vi "Power ON-Ganging.vi"(8 "error in":errorcluster, 11 "Power ON":T1={"Master/single Resource name"="", "Slave resource name"=[], "System configuration"=enum."Parallel", "Output function"=1006, "Voltage/current level"=0.0, "Voltage/current limit"=0.0, "Sense"=1009} {"Output function" items=["DC Voltage"=1006, "DC Current"=1007, "Pulse Voltage"=1049, "Pulse Current"=1050]; "Sense" items=["Local"=1008, "Remote"=1009]}) -> (0 "error out":errorcluster, 3 "Status":string)   [LabVIEW 2021]
doc: "This VI will configure the source device to DC Current or DC Voltage mode to ower on the DUT for ganged or stacked channel configuration."
uses:
  controls/Power ON-Ganging.ctl
  <instrlib>/niDCPower/nidcpower.llb/niDCPower Source Mode.ctl
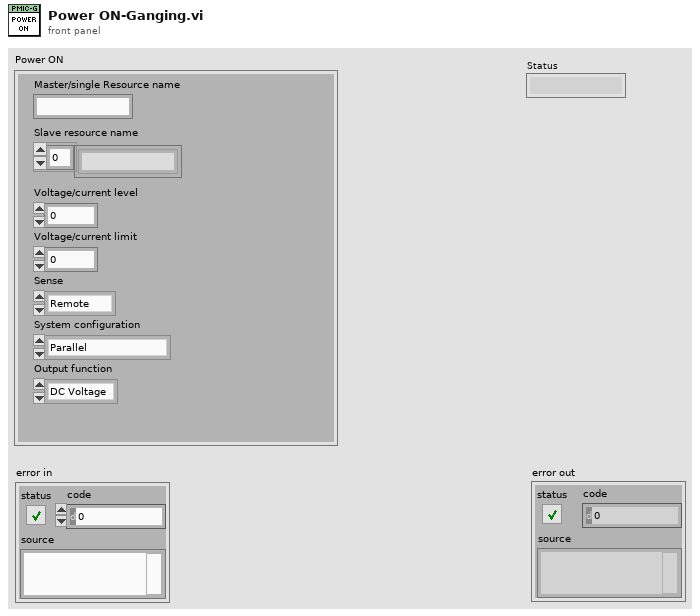
[diagram p1: front panel]
types:
  T1 = typedef "Power ON-Ganging.ctl" = cluster{"Master/single Resource name":string, "Slave resource name":string[], "System configuration":enum32{"Series", "Parallel", "Manual"}, "Output function":i32, "Voltage/current level":dbl, "Voltage/current limit":dbl, "Sense":i32}
  T2 = typedef "niDCPower Source Mode.ctl" = i32
  T3 = typedef "NIDCPower_channel_ganging - ctl - channel def.ctl" = cluster{"resource name":refnum<k15>, "channels":string, "Channel Mode":T4}
  T4 = typedef "NIDCPower_channel_ganging - ctl - channel mode.ctl" = enum32{"Master", "Slave", "Slave - Inverted"}
  T5 = typedef "NIDCPower_channel_ganging - ctl - ganged session.ctl" = cluster{"Ganged Config":T6, "Session List":refnum<k15>[], "Session Mode":T4[], "Channel":string[]}
  T6 = typedef "NIDCPower_channel_ganging - ctl - ganged config.ctl" = enum32{"Series", "Parallel", "Manual"}
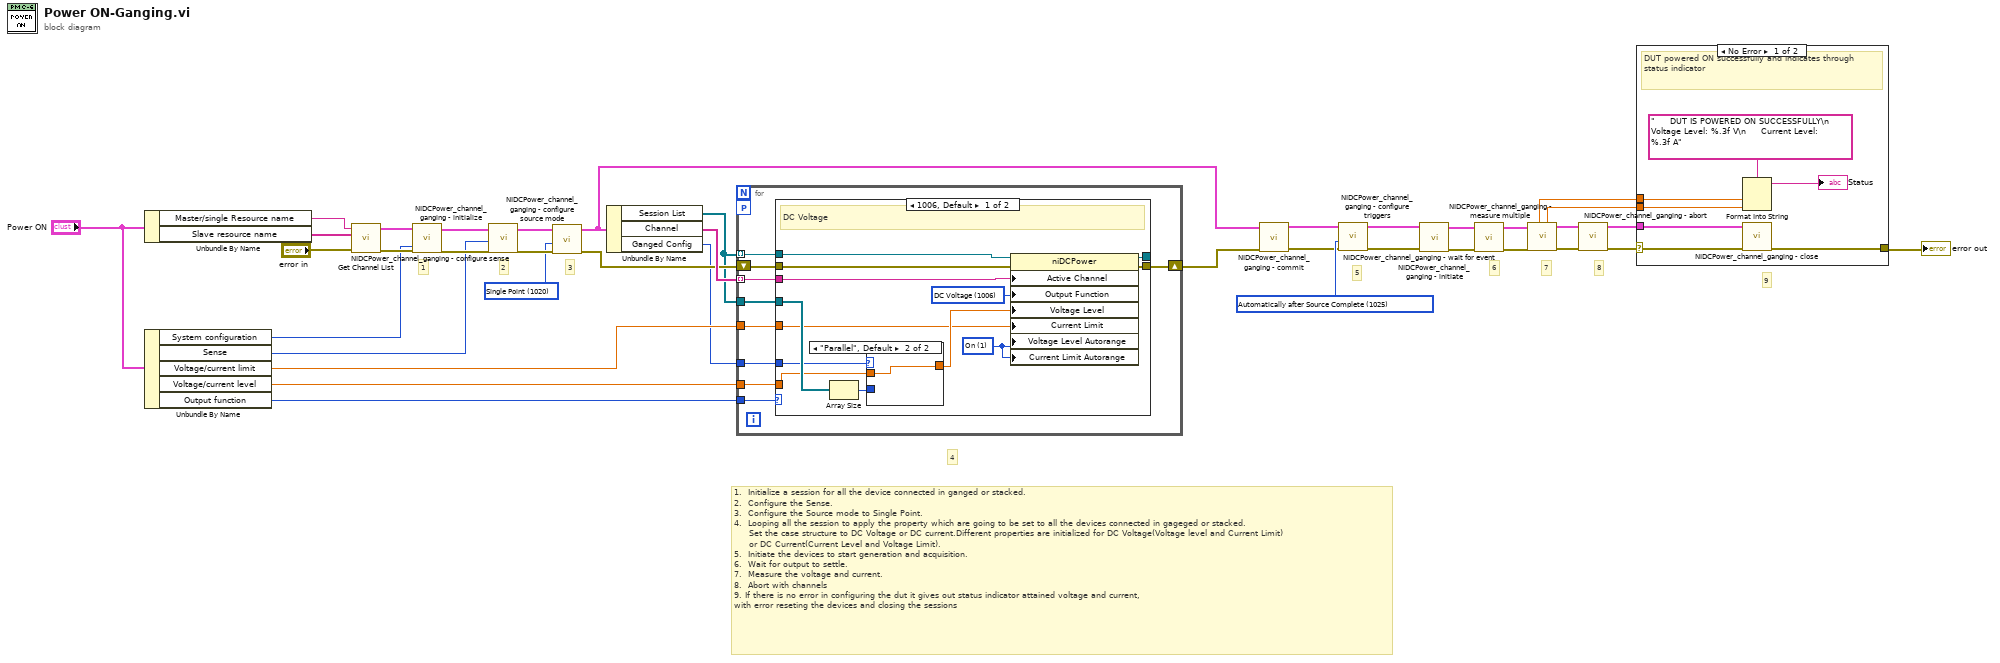
[diagram p0: block diagram]
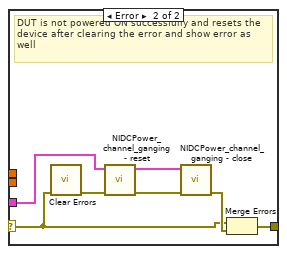
[diagram p2: hidden frame]
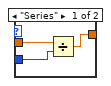
[diagram p3: hidden frame]
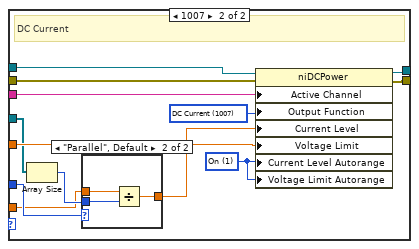
[diagram p4: hidden frame]
diagram:
  w8 = 1025 items=["Automatically after Source Complete"=1025, "On Demand"=1026, "On Measure Trigger"=1027] ("Measure When")
  w13 = T2 1020 items=["Single Point"=1020, "Sequence"=1021] ("source mode")
  # "9"
  # "8"
  # "7"
  # "6"
  # "5"
  # "4"
  # "3"
  # "2"
  # "1"
  # "1.  Initialize a session for all the device connected in ganged or stacked.\n2.  Configure the Sense.\n3.  Configure the Source mode to Single Point.\n4.  Looping all the session to apply the property which are going to be set to all the devices connected in gageged or stacked.\n     Set the case structure to DC Voltage or DC current.Different properties are initialized for DC Voltage(Voltage level and Current Limit)\n     or DC Current(Current Level and Voltage Limit). \n5.  Initiate the devices to start generation and acquisition.\n6.  Wait for output to settle.\n7.  Measure the voltage and current.\n8.  Abort with channels\n9. If there is no error in configuring the dut it gives out status indicator attained voltage and current,\nwith error reseting the devices and closing the sessions"
  n1 = Unbundle By Name("Power ON") -> ("Master/single Resource name"=w12:string, "Slave resource name"=w38:string[])
  n2 = Unbundle By Name("Power ON") -> ("System configuration"=w11:enum32{"Series", "Parallel", "Manual"}, "Sense"=w30:i32, "Voltage/current limit"=w27:dbl, "Voltage/current level"=w1:dbl, "Output function"=w10:i32)
  n3 = call "Get Channel List.vi"("error in (no error)"="error in", "Slave resource names"=w38, "Master resouce name"=w12) -> ("error out"=w35:errorcluster, "Channel List"=w36:T3[])  [unwired: 7 in]
  n4 = call "NIDCPower_channel_ganging - initialize.vi"("Ganged Config"=w11, "error in (no error)"=w35, "Channel List"=w36) -> ("error out"=w33:errorcluster, "Ganged Session Out"=w32:T5)  [unwired: 7 in]
  n5 = call "NIDCPower_channel_ganging - configure sense.vi"("error in (no error)"=w33, "sense"=w30, "Ganged Session In"=w32) -> ("error out"=w34:errorcluster, "Ganged Session Out"=w31:T5)  [unwired: 7 in]
  n6 = call "NIDCPower_channel_ganging - configure source mode.vi"("error in (no error)"=w34, "source mode"=w13, "Ganged Session In"=w31) -> ("error out"=w28:errorcluster, "Ganged Session Out"=w20:T5)  [unwired: 7 in]
  n7 = Unbundle By Name(w20) -> ("Session List"=w3:refnum<k15>[], "Channel"=w29:string[], "Ganged Config"=w2:T6)
  n8 = for {
    workers-P: _ -> [_]
    tunnel: w3 -> [w45] mode=indexing
    tunnel: w29 -> [w43] mode=indexing
    shift-right: [w42] -> w19
    shift-left: w28 -> [w44]
    tunnel: w27 -> [w46]
    tunnel: w10 -> [w47]
    tunnel: w3 -> [w41]
    tunnel: w2 -> [w40]
    tunnel: w1 -> [w39]
    n9 = case shown="1006, Default" w47 {
      tunnel: w46 -> [w48 w75]
      tunnel: w45 -> [w58 w74]
      tunnel: w44 -> [w57 w73]
      tunnel: w43 -> [w56 w72]
      tunnel: [w55 w70] -> w42
      tunnel: [w54 w71] -> _
      tunnel: w41 -> [w51 w68]
      tunnel: w40 -> [w50 w67]
      tunnel: w39 -> [w49 w65]
      frame 1006, Default {
        w59 = 1 items=["Off", "On"] ("Source:DC Voltage:Voltage Level Autorange")
        w60 = 1006 items=["DC Voltage"=1006, "DC Current"=1007, "Pulse Voltage"=1049, "Pulse Current"=1050] ("Source:Output Function")
        # "DC Voltage"
        n10 = Array Size(array=w51) -> (size(s)=w53:i32)
        n11 = case shown="\"Parallel\", Default" w50 {
          tunnel: w53 -> [w62 _]
          tunnel: w49 -> [w63 w64]
          tunnel: [w61 w64] -> w52
          frame "Series" {
            n12 = Divide(x=w63, y=w62) -> (x/y=w61:dbl)
          }
          frame "Parallel", Default {
          }
        }
        n13 = property class="niDCPower"(reference=w58, error in=w57, "Active Channel"=w56, "Output Function"=w60, "Voltage Level"=w52, "Current Limit"=w48, "Voltage Level Autorange"=w59, "Current Limit Autorange"=w59) -> (reference out=w54:refnum<k15>, error out=w55:errorcluster)
      }
      frame 1007 {
        w76 = 1 items=["Off", "On"] ("Source:DC Voltage:Voltage Level Autorange")
        w77 = 1007 items=["DC Voltage"=1006, "DC Current"=1007, "Pulse Voltage"=1049, "Pulse Current"=1050] ("Source:Output Function")
        # "DC Current"
        n14 = Array Size(array=w68) -> (size(s)=w69:i32)
        n15 = case shown="\"Parallel\", Default" w67 {
          tunnel: w65 -> [w78 w81]
          tunnel: w69 -> [_ w80]
          tunnel: [w78 w79] -> w66
          frame "Series" {
          }
          frame "Parallel", Default {
            n16 = Divide(x=w81, y=w80) -> (x/y=w79:dbl)
          }
        }
        n17 = property class="niDCPower"(reference=w74, error in=w73, "Active Channel"=w72, "Output Function"=w77, "Current Level"=w66, "Voltage Limit"=w75, "Current Level Autorange"=w76, "Voltage Limit Autorange"=w76) -> (reference out=w71:refnum<k15>, error out=w70:errorcluster)
      }
    }
  }
  n18 = call "NIDCPower_channel_ganging - commit.vi"("error in (no error)"=w19, "Ganged Session In"=w20) -> ("error out"=w7:errorcluster, "Ganged Session Out"=w5:T5)  [unwired: 8 in]
  n19 = call "NIDCPower_channel_ganging - configure triggers.vi"("error in (no error)"=w7, "Measure When"=w8, "Ganged Session In"=w5) -> ("error out"=w6:errorcluster, "Ganged Session Out"=w4:T5)  [unwired: 7 in]
  n20 = call "NIDCPower_channel_ganging - initiate.vi"("error in (no error)"=w6, "Ganged Session In"=w4) -> ("error out"=w26:errorcluster, "Ganged Session Out"=w25:T5)  [unwired: 8 in]
  n21 = call "NIDCPower_channel_ganging - wait for event.vi"("error in (no error)"=w26, "Ganged Session in"=w25) -> ("error out"=w24:errorcluster, "Ganged Session Out"=w23:T5)  [unwired: 8 in]
  n22 = call "NIDCPower_channel_ganging - measure multiple.vi"("error in (no error)"=w24, "Ganged Session In"=w23) -> ("error out"=w21:errorcluster, "Ganged Session Out"=w22:T5, "ganged current measurement"=w16:dbl, "ganged voltage measurement"=w17:dbl)  [unwired: 2 in, 4 out]
  n23 = call "NIDCPower_channel_ganging - abort.vi"("error in (no error)"=w21, "Ganged Session In"=w22) -> ("error out"=w18:errorcluster, "Ganged Session Out"=w15:T5)  [unwired: 8 in]
  n24 = case shown="No Error" w18 {
    selector: w18 -> [w84 w90]
    tunnel: w17 -> [w88 _]
    tunnel: w16 -> [w87 _]
    tunnel: w15 -> [w83 w95]
    tunnel: [w82 w89] -> w14
    frame No Error {
      # "DUT powered ON successfully and indicates through status indicator"
      n25 = Format Into String(format string="     DUT IS POWERED ON SUCCESSFULLY\n     Voltage Level: %.3f V\n     Current Level: %.3f A", w88, w87) -> (resulting string=→"Status":string)  [unwired: 2 in, 1 out]
      n26 = call "NIDCPower_channel_ganging - close.vi"("error in (no error)"=w84, "Ganged Session In"=w83) -> ("error out"=w82:errorcluster)  [unwired: 9 in]
    }
    frame Error {
      # "DUT is not powered ON successfully and resets the device after clearing the error and show error as well"
      n27 = call <vilib>:"Clear Errors.vi"("error in (no error)"=w90) -> ("error out"=w92:errorcluster)  [unwired: 5 in, 1 out]
      n28 = call "NIDCPower_channel_ganging - reset.vi"("error in (no error)"=w92, "Ganged Session In"=w95) -> ("error out"=w93:errorcluster, "Ganged Session Out"=w94:T5)  [unwired: 8 in]
      n29 = call "NIDCPower_channel_ganging - close.vi"("error in (no error)"=w93, "Ganged Session In"=w94) -> ("error out"=w91:errorcluster)  [unwired: 9 in]
      n30 = Merge Errors(w90, w91) -> (w89:errorcluster)
    }
  }
  "error out" <- w14
